vi "Receive Message.vi"(8 "error in (no error)":errorcluster, 11 "Serial Communication in":refnum<class "Serial Communication.lvclass">) -> (0 "error out":errorcluster, 3 "Serial Communication out":refnum<class "Serial Communication.lvclass">)   [LabVIEW 2018, in "Serial Communication.lvclass"]
uses:
  Serial Communication.lvclass
  Serial Communication.lvclass/Serial Communication.ctl
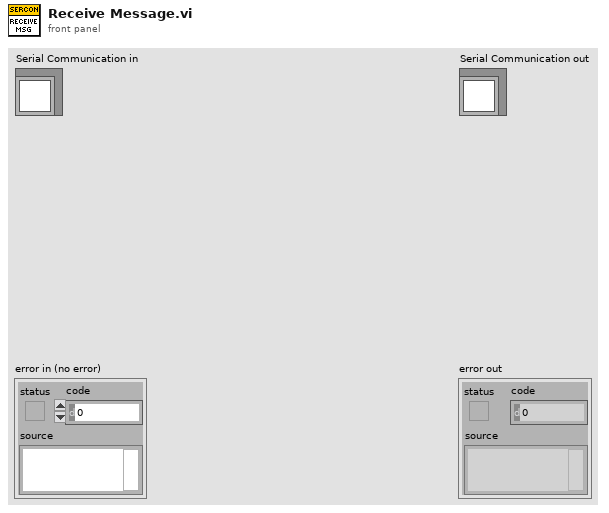
[diagram p1: front panel]
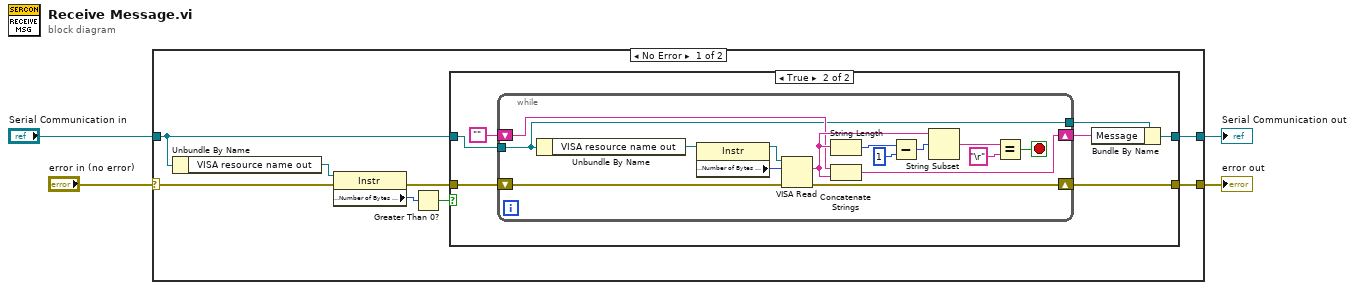
[diagram p0: block diagram]
diagram:
  n1 = case shown="No Error" "error in (no error)" {
    selector: "error in (no error)" -> [w12 w38]
    tunnel: [w10 w38] -> w2
    tunnel: "Serial Communication in" -> [w8 w37]
    tunnel: [w5 w37] -> w1
    frame No Error {
      n2 = Unbundle By Name(w8) -> ("VISA resource name out"=w7:refnum<visa-resource-name>)
      n3 = property class="Instr"(reference=w7, error in=w12) -> (error out=w11:errorcluster, "Serial Settings:Number of Bytes at Serial Port"=w6:u32)  [unwired: 1 out]
      n4 = Greater Than 0?(x=w6) -> (x > 0?=w9:bool)
      n5 = case shown="True" w9 {
        tunnel: w11 -> [w14 w21]
        tunnel: [w14 w20] -> w10
        tunnel: w8 -> [w13 w18]
        tunnel: [w13 w15] -> w5
        frame False {
        }
        frame True {
          n6 = while {
            tunnel: w18 -> [w22]
            shift-right: [w35] -> w20
            shift-left: w21 -> [w36]
            shift-right: [w23] -> w19
            shift-left: "" -> [w24]
            tunnel: [w22] -> w16
            stop <- w26 stop-if-true
            n7 = Unbundle By Name(w22) -> ("VISA resource name out"=w33:refnum<visa-resource-name>)
            n8 = property class="Instr"(reference=w33) -> (reference out=w32:refnum<visa-resource-name>, "Serial Settings:Number of Bytes at Serial Port"=w34:u32)  [unwired: 1 in, 1 out]
            n9 = VISA Read(VISA resource name=w32, byte count=w34, error in (no error)=w36) -> (read buffer=w25:string, error out=w35:errorcluster)  [unwired: 2 out]
            n10 = String Length(string=w25) -> (length=w31:i32)
            n11 = Concatenate Strings(w24, w25) -> (w23:string)
            n12 = Subtract(x=w31, y=1) -> (x-y=w29:i32)
            n13 = String Subset(string=w25, offset (0)=w29) -> (substring=w28:string)  [unwired: 1 in]
            n14 = Equal?(x=w28, y="\r") -> (x = y?=w26:bool)
          }
          n15 = Bundle By Name(cluster=w16, "Message"=w19) -> (w15:refnum<class "Serial Communication.lvclass">)
        }
      }
    }
    frame Error {
    }
  }
  "error out" <- w2
  "Serial Communication out" <- w1
